vi "Get Name.vi"(11 "Configuration in":refnum<class "Configuration.lvclass">) -> (2 "name":string, 3 "Configuration out":refnum<class "Configuration.lvclass">)   [LabVIEW 2017, in "DSF Core.lvlib" / "Configuration.lvclass"]
uses:
  Configuration.lvclass
  Configuration.lvclass/Configuration.ctl
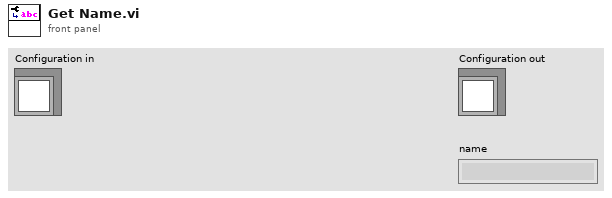
[diagram p1: front panel]
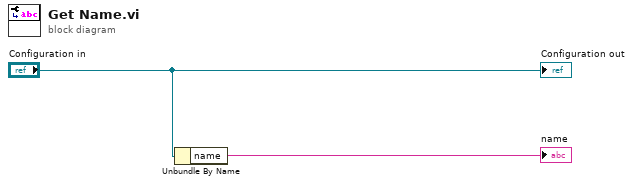
[diagram p0: block diagram]
diagram:
  n1 = Unbundle By Name("Configuration in") -> ("name"=→"name":string)
  "Configuration out" <- "Configuration in"
